vi "RPM PID loop isolated test.vi"() -> ()   [LabVIEW 2011]
uses:
  <vilib>/addons/control/pid/pid.llb/PID (DBL).vi
  <vilib>/addons/control/pid/NI_PID_pid.lvlib
panel:
  in  "ms to wait":u32
  out "dt out (s)":dbl format="%.3f"
  out "output":dbl(slide) scale=0.0..1.0
  in  "output range":cluster{"output high":dbl, "output low":dbl}={"output high"=100.0, "output low"=-100.0} {"output low" format="%.2f"; "output high" format="%.2f"}
  in  "dt (s)":dbl=-1.0 format="%.3f"
  in  "PID gains":T1={"proportional gain (Kc)"=1.0, "integral time (Ti, min)"=0.01, "derivative time (Td, min)"=0.0} {"derivative time (Td, min)" format="%.3f"; "integral time (Ti, min)" format="%.3f"; "proportional gain (Kc)" format="%.3f"}
  in  "Current RPM":dbl(slide) scale=-100.0..10000.0
  in  "RPM Setpoint":dbl
  in  "stop":bool
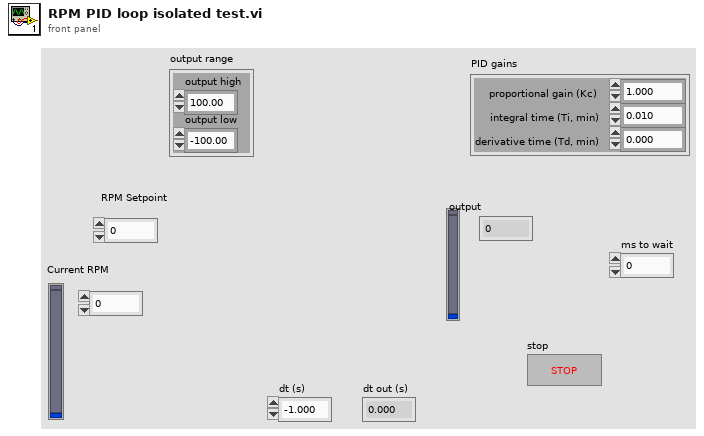
[diagram p1: front panel]
types:
  T1 = cluster{"proportional gain (Kc)":dbl, "integral time (Ti, min)":dbl, "derivative time (Td, min)":dbl}
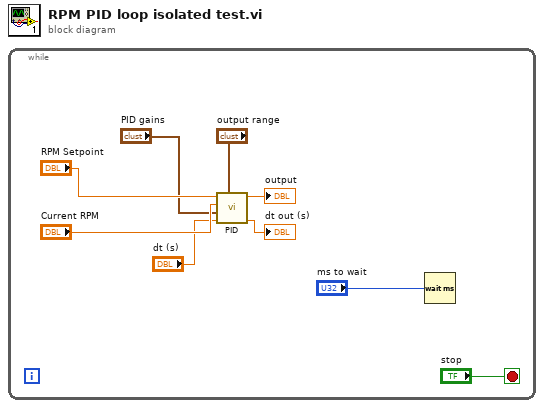
[diagram p0: block diagram]
diagram:
  n1 = while {
    stop <- "stop" stop-if-true
    n2 = call-poly <vilib>:"PID.vi"("output range"="output range", "dt (s)"="dt (s)", "PID gains"="PID gains", "process variable"="Current RPM", "setpoint"="RPM Setpoint") -> ("dt out (s)"=→"dt out (s)":dbl, "output"=→"output":dbl)  [unwired: 5 in]
    n3 = Wait (ms)(milliseconds to wait="ms to wait") -> ()  [unwired: 1 out]
  }
